vi "WSVCAP SHL FPGA LL I2C Write Data Lines.vi"(0 "Write Bit (U64)":u64, 11 "error in (no error)":errorcluster, 13 "Socket Mask":u64 format="%012x", 14 "UUT Set (0/1) (Legacy)":u8) -> (15 "error out":errorcluster)   [LabVIEW 2017]
uses:
  <vilib>/rvi/eio/common/nirviEmuTemplateMethod_errors.vi
  <vilib>/eio/EIONode/EIONode.xnode
  WSVCAP SHL FPGA LL I2C Debug Global.vi
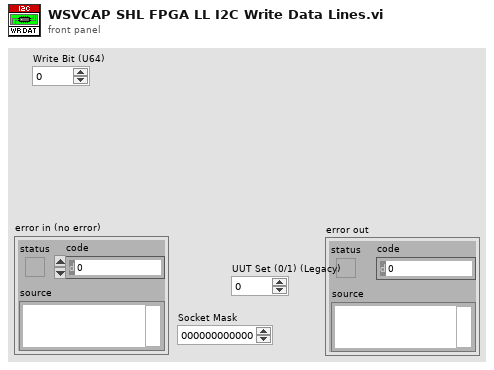
[diagram p1: front panel]
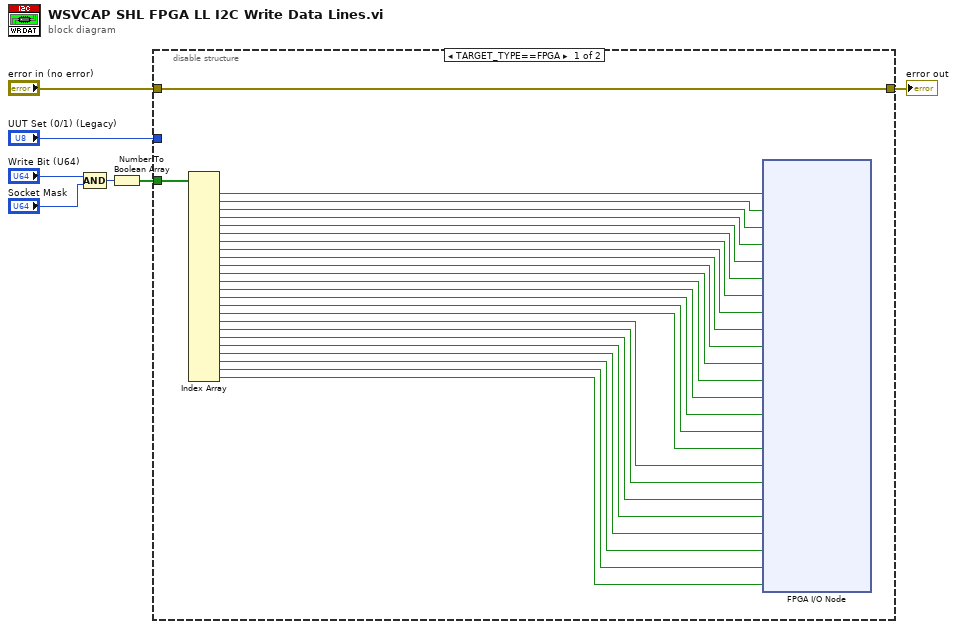
[diagram p0: block diagram]
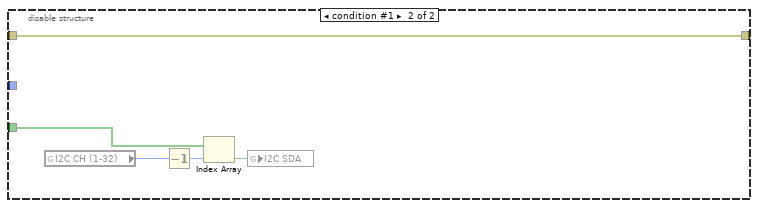
[diagram p2: hidden frame]
diagram:
  n1 = Compound Arithmetic op=AND("Write Bit (U64)", "Socket Mask") -> (w2:u64)
  n2 = Number To Boolean Array(number=w2) -> (Boolean array=w5:bool[])
  n3 = disable-structure shown="TARGET_TYPE==FPGA" {
    disable-tunnel: w5 -> [w8 w37]
    disable-tunnel: [w33 w38] -> w7
    disable-tunnel: "error in (no error)" -> [w33 w38]
    disable-tunnel: "UUT Set (0/1) (Legacy)" -> [_ _]
    frame condition #0 (active) {
      n4 = Index Array(array=w8) -> (element #1=w9:bool, element #2=w10:bool, element #3=w11:bool, element #4=w12:bool, element #5=w13:bool, element #6=w14:bool, element #7=w15:bool, element #8=w16:bool, element #9=w17:bool, element #10=w18:bool, element #11=w19:bool, element #12=w20:bool, element #13=w21:bool, element #14=w22:bool, element #15=w23:bool, element #16=w24:bool, element #17=w25:bool, element #18=w26:bool, element #19=w27:bool, element #20=w28:bool, element #21=w29:bool, element #22=w30:bool, element #23=w31:bool, element #24=w32:bool)  [unwired: 24 in]
      n5 = xnode "FPGA I/O Node"("I2C_SDA_S1"=w9, "I2C_SDA_S2"=w10, "I2C_SDA_S3"=w11, "I2C_SDA_S4"=w12, "I2C_SDA_S5"=w13, "I2C_SDA_S6"=w14, "I2C_SDA_S7"=w15, "I2C_SDA_S8"=w16, "I2C_SDA_S9"=w17, "I2C_SDA_S10"=w18, "I2C_SDA_S11"=w19, "I2C_SDA_S12"=w20, "I2C_SDA_S13"=w21, "I2C_SDA_S14"=w22, "I2C_SDA_S15"=w23, "I2C_SDA_S16"=w24, "I2C_SDA_S17"=w25, "I2C_SDA_S18"=w26, "I2C_SDA_S19"=w27, "I2C_SDA_S20"=w28, "I2C_SDA_S21"=w29, "I2C_SDA_S22"=w30, "I2C_SDA_S23"=w31, "I2C_SDA_S24"=w32) -> ()  [unwired: 25 in, 25 out]
    }
    frame condition #1 {
      n6 = global read "WSVCAP SHL FPGA LL I2C Debug Global.vi" "I2C CH (1-32)"() -> (w36:i32)
      n7 = Decrement(x=w36) -> (x-1=w34:i32)
      n8 = Index Array(array=w37, index=w34) -> (element=w35:bool)
      n9 = global write "WSVCAP SHL FPGA LL I2C Debug Global.vi" "I2C SDA"(w35) -> ()
    }
  }
  "error out" <- w7
